vi "Proiect.vi"() -> ()   [LabVIEW 2026]
uses:
  <vilib>/Utility/miscctls.llb/LVBoundsTypeDef.ctl
panel:
  in  "Input":bool[][](array[boolean])
  out "State":string[][](array[string])
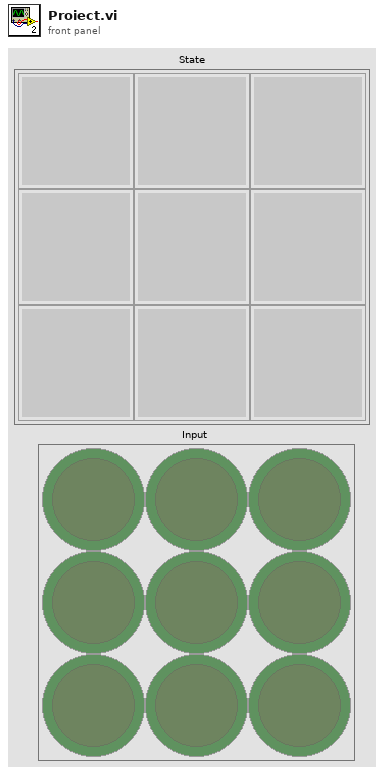
[diagram p1: front panel]
types:
  T1 = typedef "LVBoundsTypeDef.ctl" = cluster{"Width":u32, "Height":u32}
  T2 = enum16{"None", "Stacked", "Clockwise", "Counterclockwise"}
  T3 = enum16{"Init", "PlayerMove", "PcMove", "CheckWinUser", "CheckWinPc", "Draw", "YouWin", "GameOver", "Exit"}
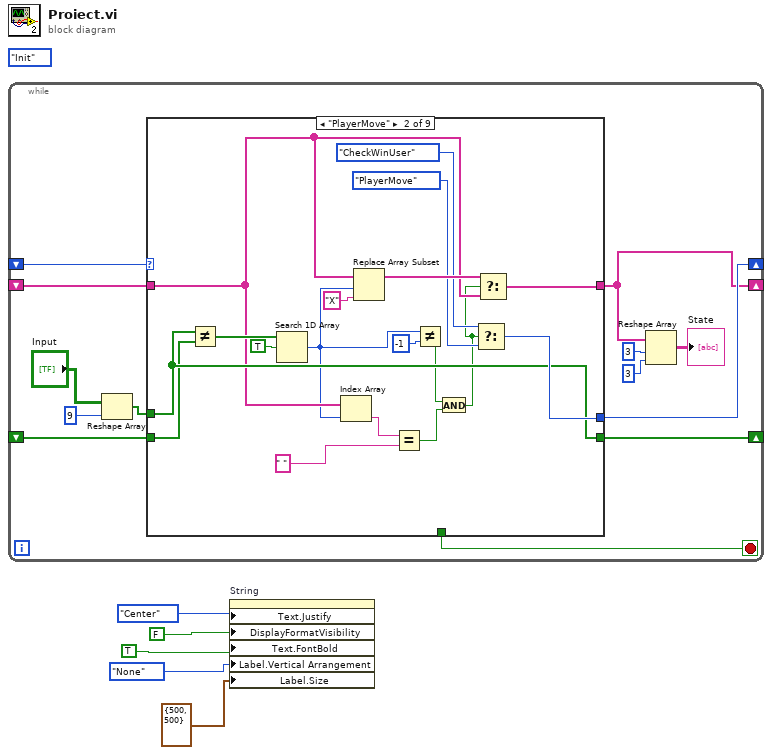
[diagram p0: block diagram]
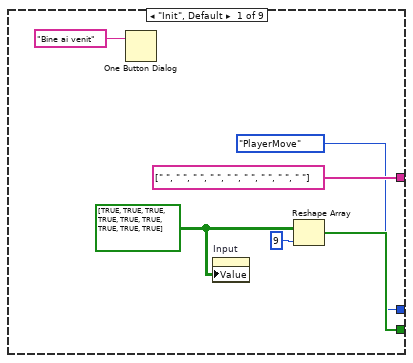
[diagram p2: hidden frame]
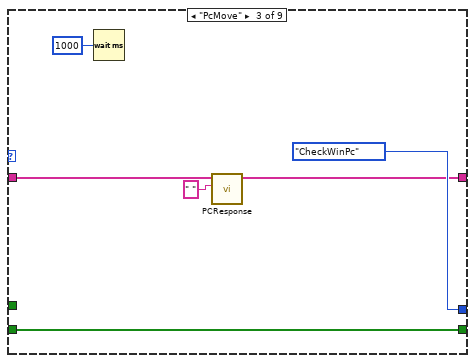
[diagram p3: hidden frame]
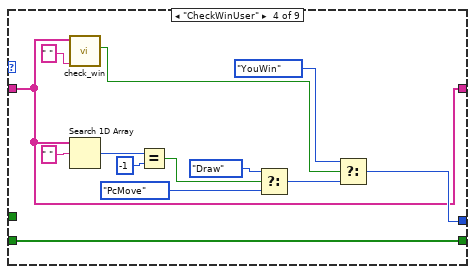
[diagram p4: hidden frame]
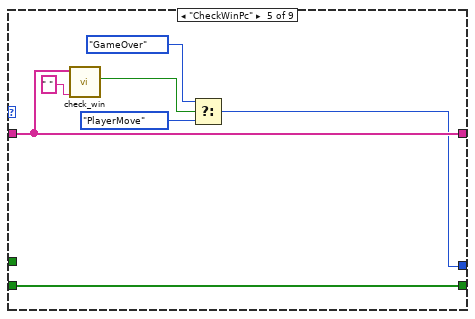
[diagram p5: hidden frame]
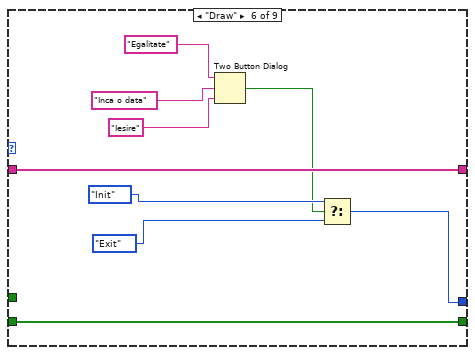
[diagram p6: hidden frame]
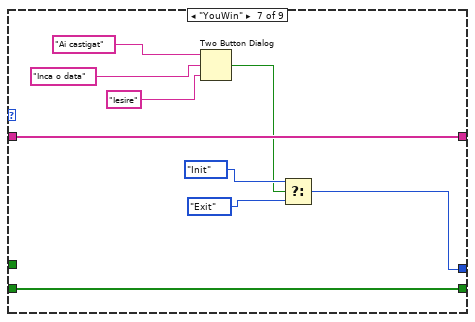
[diagram p7: hidden frame]
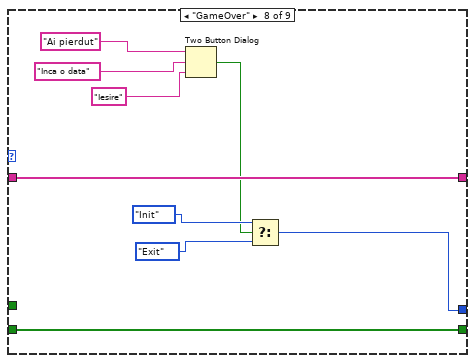
[diagram p8: hidden frame]
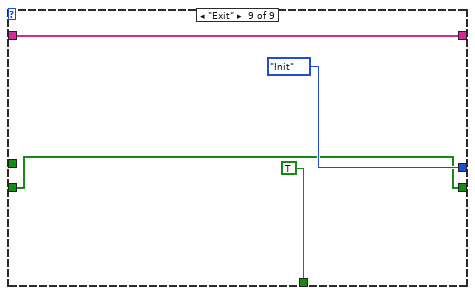
[diagram p9: hidden frame]
diagram:
  (unwired) T3."Init"
  n1 = while {
    shift-right: [w17] -> _
    shift-left: _ -> [w18]
    shift-right: [w9] -> _
    shift-left: _ -> [w8]
    shift-right: [w16] -> _
    shift-left: _ -> [w15]
    stop <- w7 stop-if-true
    n2 = Reshape Array("Input", 9 ("dimension size")) -> (w13:bool[])
    n3 = case shown="\"PlayerMove\"" w18 {
      tunnel: [T3."PlayerMove" w41 T3."CheckWinPc" w58 w62 w69 w78 w87 T3."Init"] -> w17
      tunnel: [string[] [" ", " ", " ", " ", " ", " ", " ", " ", " "] w38 w45 w56 w63 w77 w86 w95 w97] -> w9
      tunnel: w13 -> [_ w35 _ _ _ _ _ _ _]
      tunnel: [w21 w35 w48 w61 w68 w76 w85 w94 w96] -> w16
      tunnel: w15 -> [_ w34 w48 w61 w68 w76 w85 w94 w96]
      tunnel: w8 -> [_ w30 w46 w56 w63 w77 w86 w95 w97]
      tunnel: [_ _ _ _ _ _ _ _ TRUE] -> w7
      frame "Init", Default {
        w19 = bool[][] [[TRUE, TRUE, TRUE], [TRUE, TRUE, TRUE], [TRUE, TRUE, TRUE]] ("Array 2")
        n4 = One Button Dialog(message="Bine ai venit") -> ()  [unwired: 1 in, 1 out]
        n5 = property on="Input" class="Arr (strict)"("Value"=w19) -> ()  [unwired: 2 in, 2 out]
        n6 = Reshape Array(w19, 9 ("dimension size")) -> (w21:bool[])
      }
      frame "PlayerMove" {
        n7 = Not Equal?(x=w35, y=w34) -> (x != y?=w40:bool[])
        n8 = Search 1D Array(1D array=w40, element=TRUE) -> (index of element=w29:i32)  [unwired: 1 in]
        n9 = Index Array(array=w30, index=w29) -> (element=w28:string)
        n10 = Replace Array Subset(array=w30, new element="X" ("new element/subarray"), index=w29) -> (w36:string[])
        n11 = Equal?(x=w28, y=" ") -> (x = y?=w25:bool)
        n12 = Not Equal?(x=w29, y=-1) -> (x != y?=w26:bool)
        n13 = And(x=w26, y=w25) -> (x .and. y?=w27:bool)
        n14 = Select(t=T3."CheckWinUser", s=w27, f=T3."PlayerMove") -> (s? t:f=w41:T3)
        n15 = Select(t=w36, s=w27, f=w30) -> (s? t:f=w38:string[])
      }
      frame "PcMove" {
        n16 = Wait (ms)(milliseconds to wait=u32 1000) -> ()  [unwired: 1 out]
        n17 = call "PCResponse.vi"("String"=" ", "Array"=w46) -> ("Array 2"=w45:string[])  [unwired: 8 in, 1 out]
      }
      frame "CheckWinUser" {
        n18 = call "check_win.vi"("check against"=" ", "Array"=w56) -> ("result"=w59:bool)  [unwired: 9 in]
        n19 = Search 1D Array(1D array=w56, element=" ") -> (index of element=w54:i32)  [unwired: 1 in]
        n20 = Equal?(x=w54, y=-1) -> (x = y?=w50:bool)
        n21 = Select(t=T3."Draw", s=w50, f=T3."PcMove") -> (s? t:f=w49:T3)
        n22 = Select(t=T3."YouWin", s=w59, f=w49) -> (s? t:f=w58:T3)
      }
      frame "CheckWinPc" {
        n23 = call "check_win.vi"("check against"=" ", "Array"=w63) -> ("result"=w66:bool)  [unwired: 9 in]
        n24 = Select(t=T3."GameOver", s=w66, f=T3."PlayerMove") -> (s? t:f=w62:T3)
      }
      frame "Draw" {
        n25 = Two Button Dialog(message="Egalitate", 1:"Iesire" ("F button name (\"Cancel\")"), 2:"Inca o data" ("T button name (\"OK\")")) -> (T button?=w70:bool)
        n26 = Select(t=T3."Init", s=w70, f=T3."Exit") -> (s? t:f=w69:T3)
      }
      frame "YouWin" {
        n27 = Two Button Dialog(message="Ai castigat", 1:"Iesire" ("F button name (\"Cancel\")"), 2:"Inca o data" ("T button name (\"OK\")")) -> (T button?=w79:bool)
        n28 = Select(t=T3."Init", s=w79, f=T3."Exit") -> (s? t:f=w78:T3)
      }
      frame "GameOver" {
        n29 = Two Button Dialog(message="Ai pierdut", 1:"Iesire" ("F button name (\"Cancel\")"), 2:"Inca o data" ("T button name (\"OK\")")) -> (T button?=w88:bool)
        n30 = Select(t=T3."Init", s=w88, f=T3."Exit") -> (s? t:f=w87:T3)
      }
      frame "Exit" {
      }
    }
    n31 = Reshape Array(w9, 3 ("dimension size"), 3 ("dimension size")) -> (→"State":string[][])
  }
  n32 = property on="String" class="Str"("Text.Justify"=enum16{"Left", "Center", "Right"}."Center" ("Text.Justification"), "DisplayFormatVisibility"=FALSE ("Text.Size to Text?"), "Text.FontBold"=TRUE ("Text.Font:Bold"), "Label.Vertical Arrangement"=T2."None", "Label.Size"=T1 {"Width"=500, "Height"=500}) -> ()  [unwired: 2 in, 2 out]
